vi "AddUser-Windows.vi"(7 "Login-UI.lvlib:PwdMgr.lvclass":refnum<class "PwdMgr.lvclass">, 8 "error in":errorcluster) -> (0 "error out":errorcluster)   [LabVIEW 2020, in "Login-UI.lvlib"]
uses:
  Login-UI.lvlib
  _Typedef/User-Role.ctl
  PwdMgr/PwdMgr.lvclass
  _Typedef/User-Info.ctl
panel:
  in  "Exit":bool
  in  "Save":bool
  in  "权  限":T1
  in  "密  码":string
  in  "用户名":string
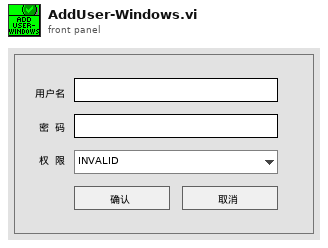
[diagram p1: front panel]
types:
  T1 = typedef "Login-UI.lvlib/User-Role.ctl" = enum16{"INVALID", "Operator", "Engineer", "Admin", "Anonymous"}
  T2 = enum32{"Invalid", "Standard", "Closed", "Hidden", "Minimized", "Maximized"}
  T3 = enum32{"invalid app kind", "Development System", "Run Time System", "Student Edition", "Embedded LabVIEW", "Evaluation", "Custom"}
  T4 = typedef "Login-UI.lvlib/User-Info.ctl" = cluster{"UserName":string, "Password":string, "Role":T1}
  T5 = cluster{"Core":cluster{"Current VI Reference":refnum<vi>, "Close Panel on Exit?":bool}, "Your Boolean data":bool, "Your string data":string, "Cluster":T4}
  T6 = typedef "eventvkey.ctl" = enum16{"ASCII", "Enter", "Return", "Shift", "Ctrl", "Alt", "Cmd", "Opt", "Caps", "NumLock", "Clear", "Break", "Up", "Down", "Left", "Right", "Insert", "Delete", "Home", "End", "PageUp", "PageDown", "Escape", "Help", "Pause", "ScrollLock", "F1", "F2", "F3", "F4", "F5", "F6", "F7", "F8", "F9", "F10", "F11", "F12", "F13", "F14", "F15", "F16", "F17", "F18", "F19", "F20", "F21", "F22", "F23", "F24", "Play", "VolumeUp", "VolumeDown", "Mute", "Two Byte Char"}
  T7 = cluster{"Current VI Reference":refnum<vi>, "Close Panel on Exit?":bool}
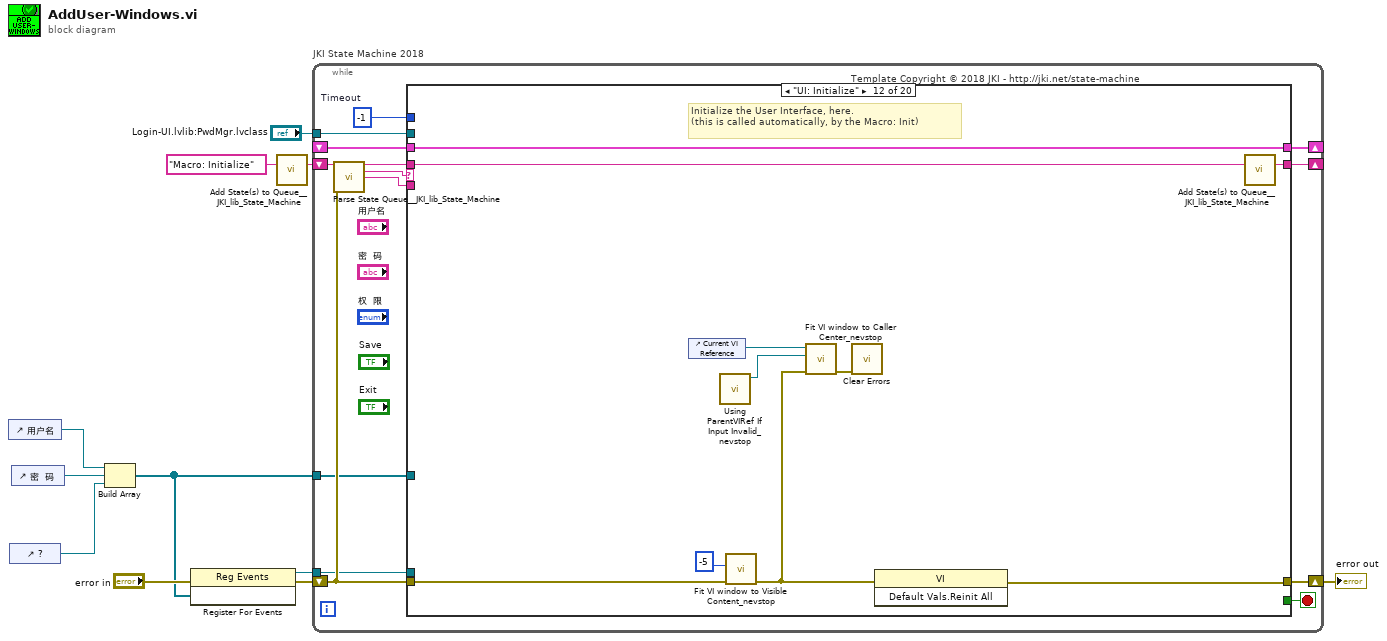
[diagram p0: block diagram]
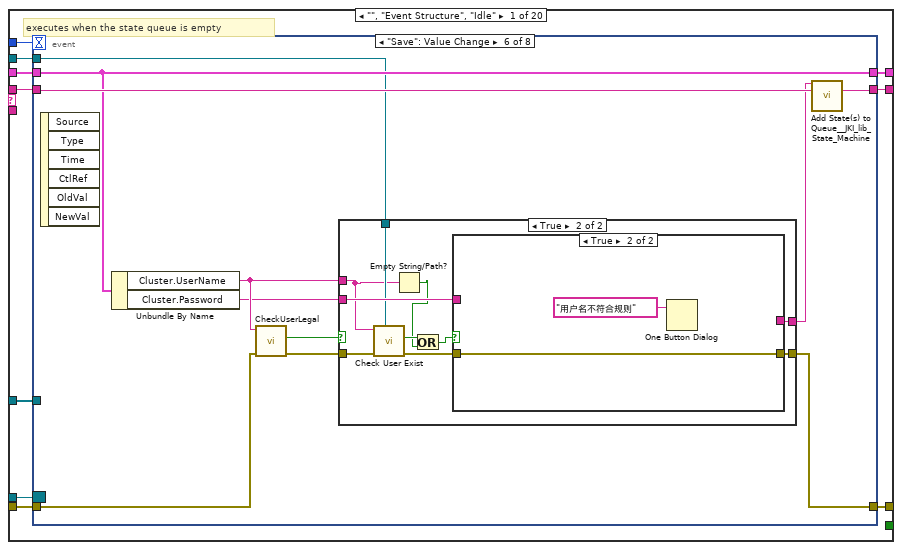
[diagram p2: hidden frame]
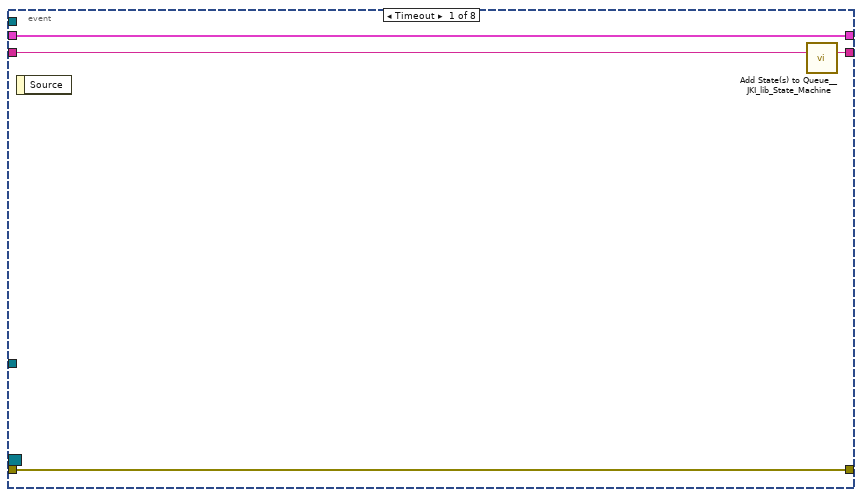
[diagram p3: hidden frame]
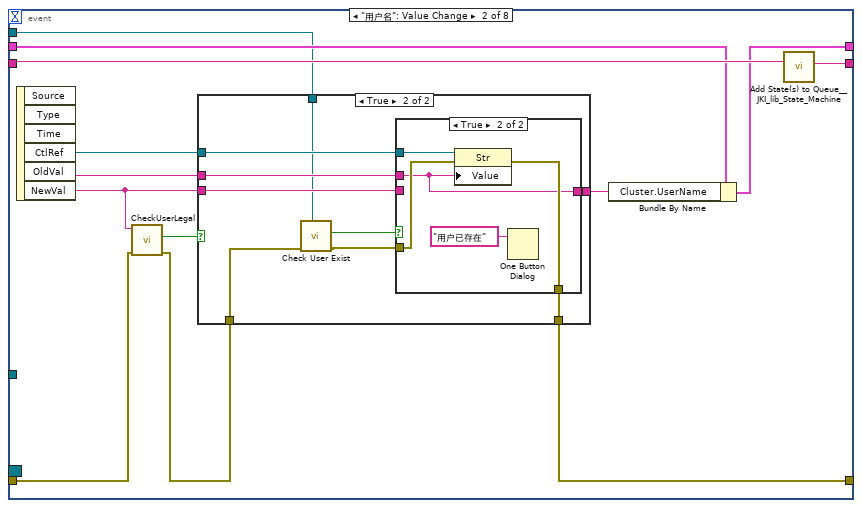
[diagram p4: hidden frame]
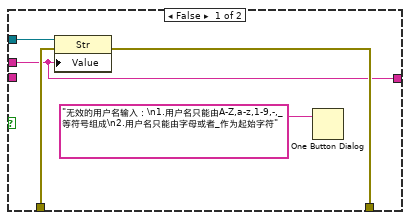
[diagram p5: hidden frame]
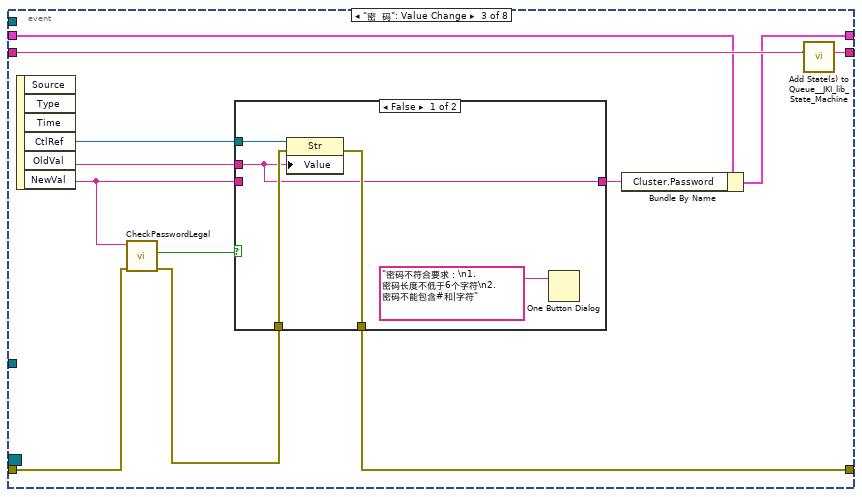
[diagram p7: hidden frame]
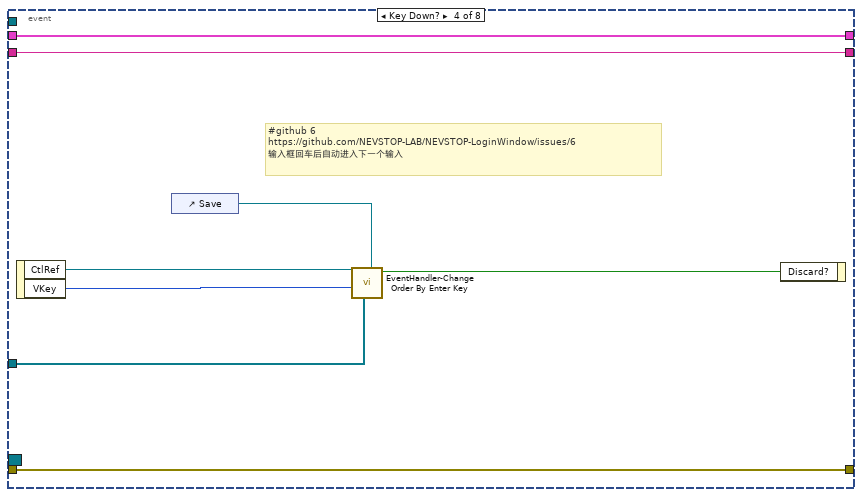
[diagram p9: hidden frame]
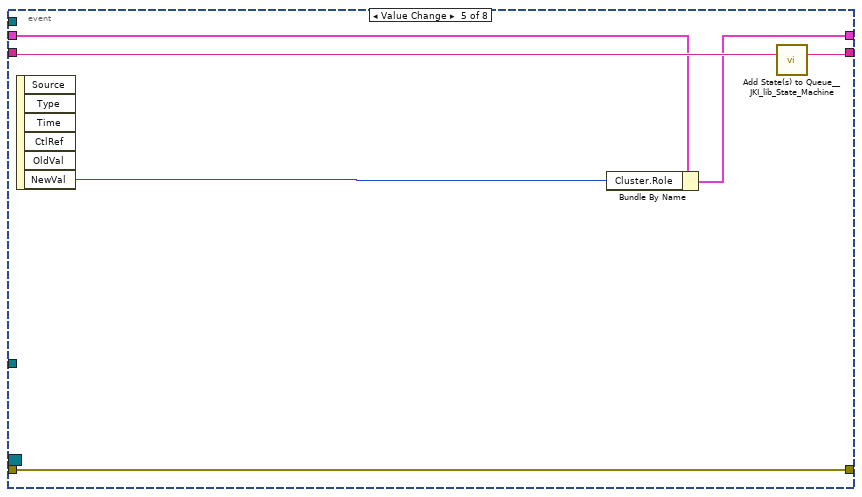
[diagram p10: hidden frame]
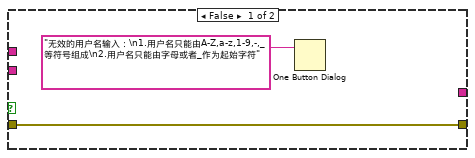
[diagram p11: hidden frame]
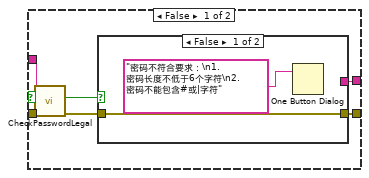
[diagram p12: hidden frame]
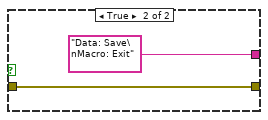
[diagram p13: hidden frame]
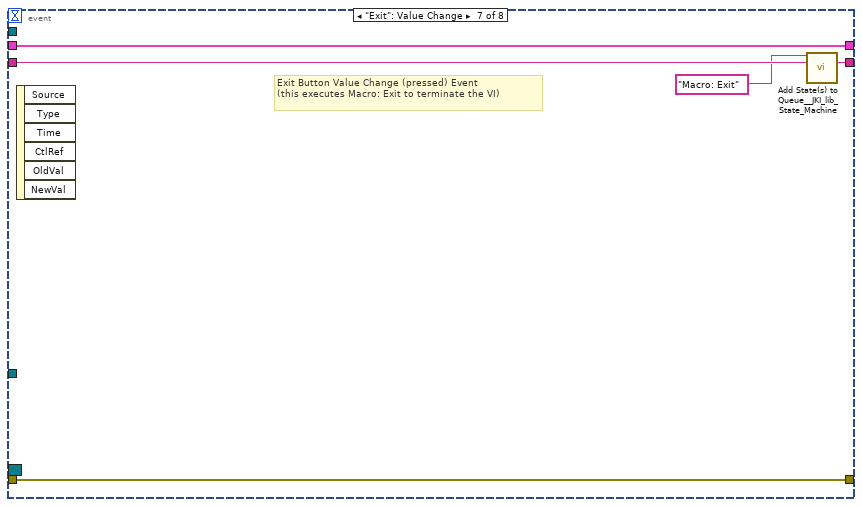
[diagram p14: hidden frame]
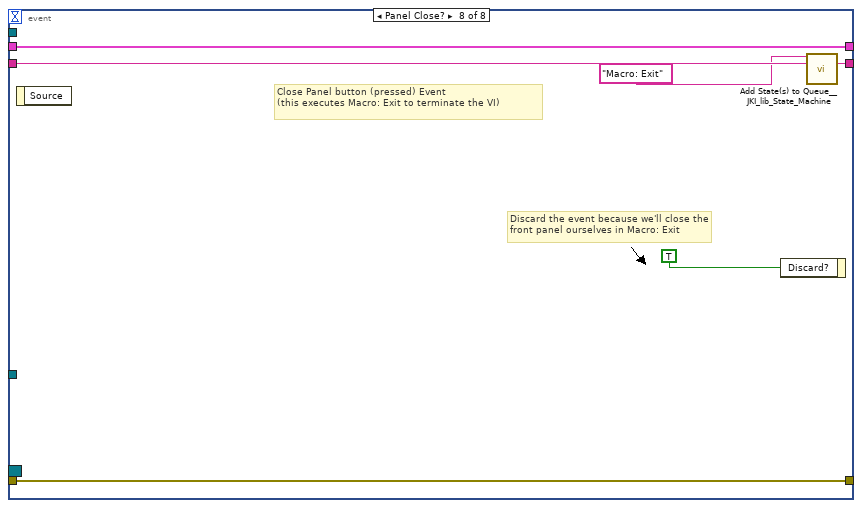
[diagram p15: hidden frame]
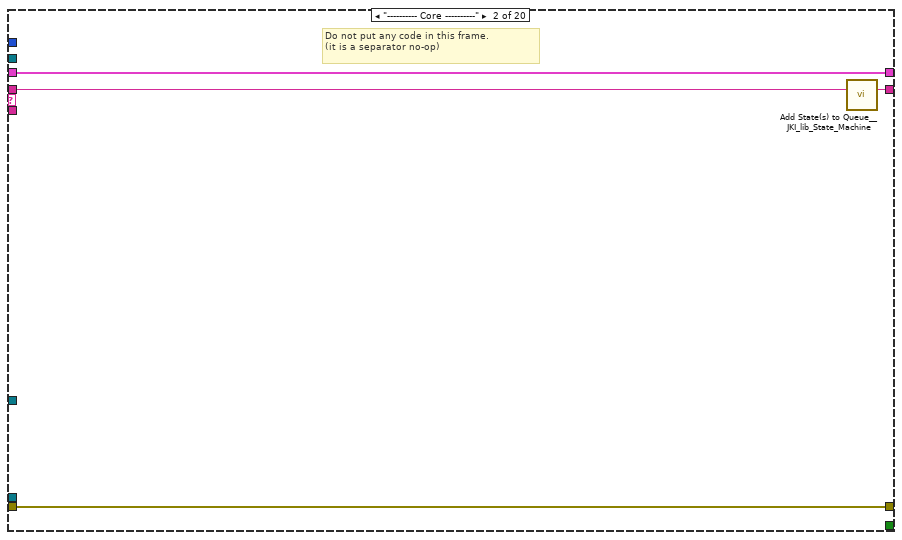
[diagram p16: hidden frame]
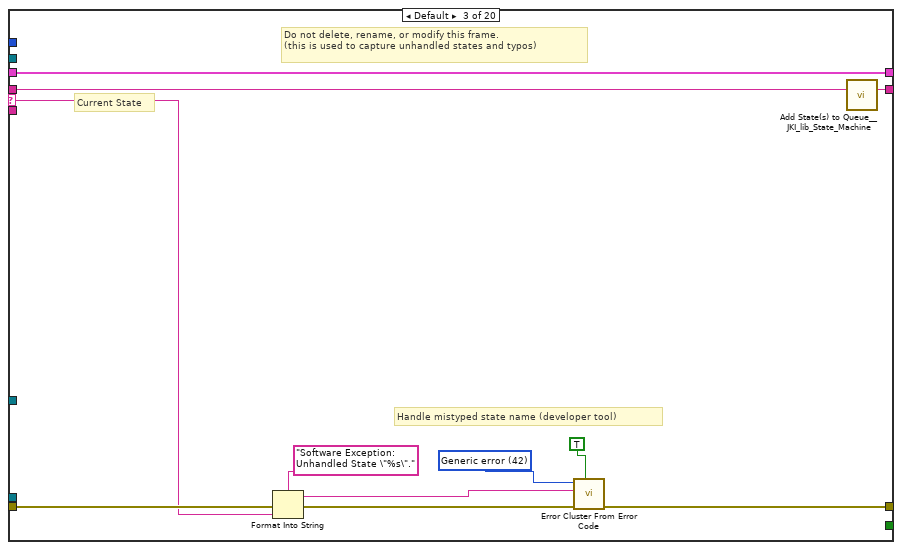
[diagram p17: hidden frame]
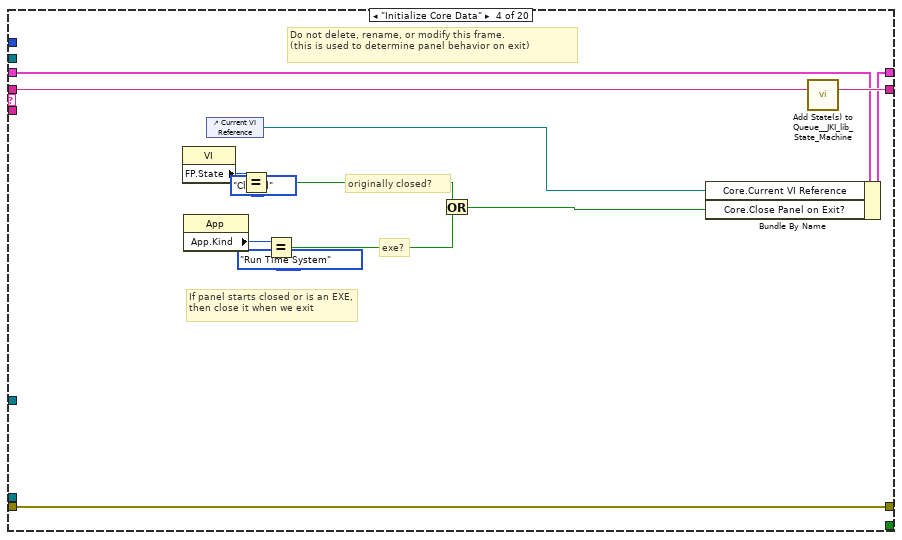
[diagram p18: hidden frame]
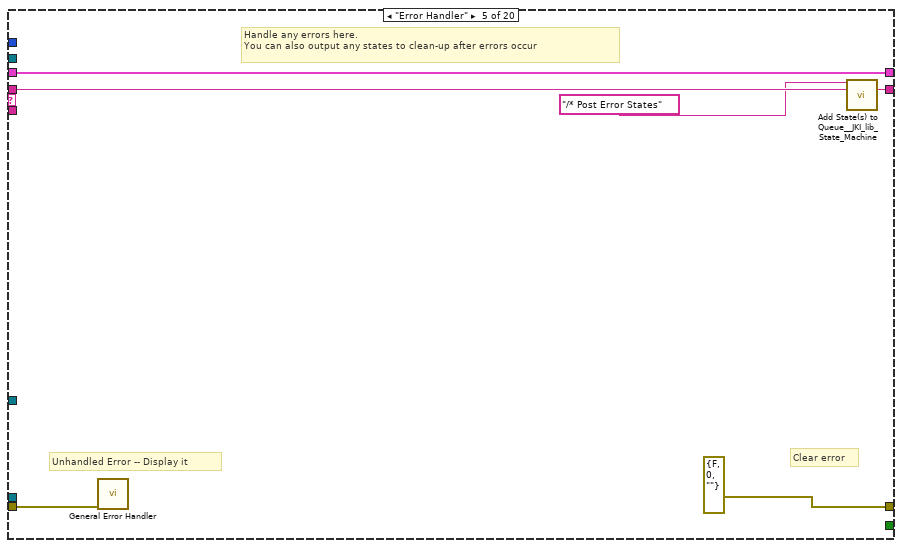
[diagram p19: hidden frame]
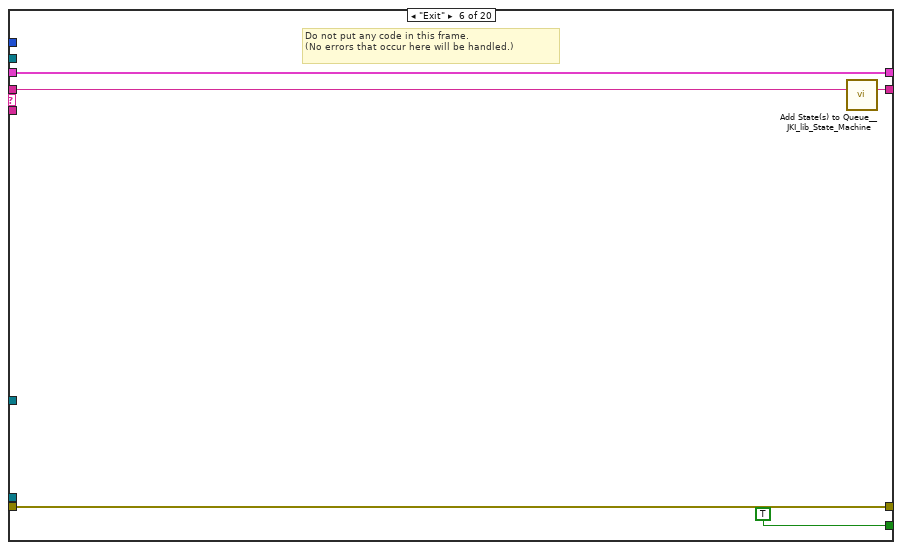
[diagram p20: hidden frame]
diagram:
  n1 = control-ref of="用户名"() -> (w2:refnum<vi>)
  n2 = control-ref of="?"() -> (w7:refnum<vi>)
  n3 = control-ref of="密  码"() -> (w3:refnum<vi>)
  n4 = Build Array(w2, w3, w7) -> (w4:refnum<vi>[])
  n5 = register-events(error in="error in", w4) -> (reference out=w5:refnum<event-registration>, error out=w6:errorcluster)  [unwired: 1 in]
  n6 = call <vilib>:"Add State(s) to Queue__JKI_lib_State_Machine.vi"("State(s) in (\"\")"="Macro: Initialize") -> ("States Out"=w11:string)  [unwired: 14 in]
  n7 = while "JKI State Machine 2018" {
    shift-right: [w18] -> _
    shift-left: _ -> [w17]
    shift-right: [w21] -> w8
    shift-left: w6 -> [w15]
    shift-right: [w20] -> _
    shift-left: w11 -> [w22]
    tunnel: w5 -> [w14]
    tunnel: w4 -> [w13]
    tunnel: "Login-UI.lvlib:PwdMgr.lvclass" -> [w12]
    stop <- w19 stop-if-true
    w16 = -1  # Timeout
    # "Template Copyright © 2018 JKI - http://jki.net/state-machine"
    n8 = call <vilib>:"Parse State Queue__JKI_lib_State_Machine.vi"("State Queue"=w22, "Error In (no error)"=w15) -> ("Remaining States"=w24:string, "Current State"=w25:string, "Arguments"=w23:string)  [unwired: 11 in]
    n9 = case shown="\"UI: Initialize\"" w25 {
      selector: w25 -> [_ _ w157 _ _ _ _ _ _ _ _ _ _ _ _ _ _ _ _ _]
      tunnel: w24 -> [w35 w156 w161 w180 w186 w191 w195 w203 w212 w219 w223 w233 w239 w250 w319 w324 w334 w338 w342 w346]
      tunnel: w23 -> [_ _ _ _ _ _ _ _ _ _ _ _ w234 w244 _ _ _ _ _ _]
      tunnel: w17 -> [w34 w153 w159 w173 w183 w189 w192 _ w210 w214 w220 w231 w237 w246 w316 w321 w331 w335 w339 w343]
      tunnel: [w33 w154 w163 w177 errorcluster {"status"=FALSE, "code"=0, "source"=""} ("error out") w188 w193 w200 w205 w215 w221 w228 w235 w247 w317 w322 w332 w336 w340 w344] -> w21
      tunnel: w15 -> [w32 w154 w162 w177 w182 w188 w193 w200 w207 w216 w221 w229 w236 w248 w317 w322 w332 w336 w340 w344]
      tunnel: [w29 w155 w160 w179 w185 w190 w194 w202 w213 w218 w222 w232 w238 w249 w318 w323 w333 w337 w341 w345] -> w20
      tunnel: [_ _ _ _ _ TRUE _ _ _ _ _ _ _ _ _ _ _ _ _ _] -> w19
      tunnel: [w31 w153 w159 w178 w183 w189 w192 w201 w210 w214 w220 w231 w237 w246 w316 w321 w331 w335 w339 w343] -> w18
      tunnel: w16 -> [w30 _ _ _ _ _ _ _ _ _ _ _ _ _ _ _ _ _ _ _]
      tunnel: w14 -> [w28 _ _ _ _ _ _ _ _ _ _ _ _ _ _ _ _ _ _ _]
      tunnel: w13 -> [w27 _ _ _ _ _ _ _ _ _ _ _ _ _ _ _ _ _ _ _]
      tunnel: w12 -> [w26 _ _ _ _ _ _ _ w204 _ _ _ _ _ _ _ _ _ _ _]
      frame "", "Event Structure", "Idle" {
        # "executes when the state queue is empty"
        n10 = event shown="[5] \"Save\": Value Change" {
          selector: w28 -> [_ _ _ _ _ _ _ _]
          dyn-events: _ -> [_ _ _ _ _ _ _ _]
          timeout: w30 -> [_ _ _ _ _ _ _ _]
          tunnel: w35 -> [w39 w48 w81 w94 w104 w116 w146 w152]
          tunnel: [w38 w49 w82 w94 w105 w117 w145 w151] -> w29
          tunnel: w34 -> [w36 w43 w76 w95 w102 w112 w143 w149]
          tunnel: [w37 w50 w83 w93 w106 w108 w144 w150] -> w33
          tunnel: w32 -> [w37 w45 w79 w93 w106 w109 w144 w150]
          tunnel: [w36 w41 w74 w95 w101 w112 w143 w149] -> w31
          tunnel: w27 -> [_ _ _ w97 _ _ _ _]
          tunnel: w26 -> [_ w40 _ _ _ w107 _ _]
          event Timeout {
            n11 = event-data() -> ()  [unwired: 1 in, 1 out]
            n12 = call <vilib>:"Add State(s) to Queue__JKI_lib_State_Machine.vi"("State(s) in (\"\")"=w39) -> ("States Out"=w38:string)  [unwired: 14 in]
          }
          event "用户名": Value Change {
            n13 = event-data() -> ("CtlRef"=w52:refnum<vi>, "OldVal"=w51:string, "NewVal"=w46:string)  [unwired: 1 in, 3 out]
            n14 = call "CheckUserLegal.vi"("error in (no error)"=w45, "Username"=w46) -> ("error out"=w44:errorcluster, "Legal?"=w47:bool)  [unwired: 8 in]
            n15 = case shown="True" w47 {
              tunnel: w52 -> [w56 w66]
              tunnel: w51 -> [w53 w65]
              tunnel: w46 -> [_ w60]
              tunnel: w44 -> [w55 w62]
              tunnel: [w54 w64] -> w50
              tunnel: [w53 w59] -> w42
              tunnel: w40 -> [_ w58]
              frame False {
                n16 = property class="Str"(reference=w56, error in=w55, "Value"=w53) -> (error out=w54:errorcluster)  [unwired: 1 out]
                n17 = One Button Dialog(message="无效的用户名输入：\n1.用户名只能由A-Z,a-z,1-9,-,_等符号组成\n2.用户名只能由字母或者_作为起始字符") -> ()  [unwired: 1 in, 1 out]
              }
              frame True {
                n18 = call-dynamic "Check User Exist.vi"("PwdMgr in"=w58, "Error in"=w62) -> ("Error out"=w61:errorcluster, "exist？"=w63:bool)  [unwired: 7 in, 1 out]
                n19 = case shown="True" w63 {
                  tunnel: w66 -> [_ w72]
                  tunnel: w65 -> [_ w69]
                  tunnel: w61 -> [w68 w71]
                  tunnel: [w68 w70] -> w64
                  tunnel: [w67 w69] -> w59
                  tunnel: w60 -> [w67 _]
                  frame False {
                  }
                  frame True {
                    n20 = property class="Str"(reference=w72, error in=w71, "Value"=w69) -> (error out=w70:errorcluster)  [unwired: 1 out]
                    n21 = One Button Dialog(message="用户已存在") -> ()  [unwired: 1 in, 1 out]
                  }
                }
              }
            }
            n22 = Bundle By Name(cluster=w43, "Cluster.UserName"=w42) -> (w41:T5)
            n23 = call <vilib>:"Add State(s) to Queue__JKI_lib_State_Machine.vi"("State(s) in (\"\")"=w48) -> ("States Out"=w49:string)  [unwired: 14 in]
          }
          event "密  码": Value Change {
            n24 = event-data() -> ("CtlRef"=w84:refnum<vi>, "OldVal"=w85:string, "NewVal"=w80:string)  [unwired: 1 in, 3 out]
            n25 = call "CheckPasswordLegal.vi"("error in (no error)"=w79, "Password"=w80) -> ("error out"=w78:errorcluster, "legal?"=w77:bool)  [unwired: 8 in]
            n26 = case shown="False" w77 {
              tunnel: w85 -> [w86 _]
              tunnel: w80 -> [_ w91]
              tunnel: [w89 w92] -> w83
              tunnel: w84 -> [w88 _]
              tunnel: w78 -> [w87 w92]
              tunnel: [w86 w91] -> w75
              frame False {
                n27 = property class="Str"(reference=w88, error in=w87, "Value"=w86) -> (error out=w89:errorcluster)  [unwired: 1 out]
                n28 = One Button Dialog(message="密码不符合要求：\n1.密码长度不低于6个字符\n2. 密码不能包含#和|字符") -> ()  [unwired: 1 in, 1 out]
              }
              frame True {
              }
            }
            n29 = Bundle By Name(cluster=w76, "Cluster.Password"=w75) -> (w74:T5)
            n30 = call <vilib>:"Add State(s) to Queue__JKI_lib_State_Machine.vi"("State(s) in (\"\")"=w81) -> ("States Out"=w82:string)  [unwired: 14 in]
          }
          event Key Down? {
            # "#github 6\nhttps://github.com/NEVSTOP-LAB/NEVSTOP-LoginWindow/issues/6\n输入框回车后自动进入下一个输入"
            n31 = event-data() -> ("CtlRef"=w100:refnum<vi>, "VKey"=w99:T6)  [unwired: 1 in]
            n32 = control-ref of="Save"() -> (w98:refnum<vi>)
            n33 = call "EventHandler-Change Order By Enter Key.vi"("Next Ctrl"=w98, "Controls for changing order"=w97, "VKey"=w99, "Event Control"=w100) -> ("Discard?"=w96:bool)  [unwired: 7 in]
            n34 = event-data("Discard?"=w96) -> ()  [unwired: 1 in, 1 out]
          }
          event Value Change {
            n35 = event-data() -> ("NewVal"=w103:T1)  [unwired: 1 in, 5 out]
            n36 = Bundle By Name(cluster=w102, "Cluster.Role"=w103) -> (w101:T5)
            n37 = call <vilib>:"Add State(s) to Queue__JKI_lib_State_Machine.vi"("State(s) in (\"\")"=w104) -> ("States Out"=w105:string)  [unwired: 14 in]
          }
          event "Save": Value Change {
            n38 = event-data() -> ()  [unwired: 1 in, 6 out]
            n39 = Unbundle By Name(w112) -> ("Cluster.UserName"=w114:string, "Cluster.Password"=w113:string)
            n40 = call "CheckUserLegal.vi"("error in (no error)"=w109, "Username"=w114) -> ("error out"=w110:errorcluster, "Legal?"=w115:bool)  [unwired: 8 in]
            n41 = case shown="True" w115 {
              tunnel: w114 -> [_ w122]
              tunnel: w113 -> [_ w128]
              tunnel: [_ w127] -> w111
              tunnel: w110 -> [w119 w126]
              tunnel: [w119 w124] -> w108
              tunnel: w107 -> [_ w123]
              frame False {
                n42 = One Button Dialog(message="无效的用户名输入：\n1.用户名只能由A-Z,a-z,1-9,-,_等符号组成\n2.用户名只能由字母或者_作为起始字符") -> ()  [unwired: 1 in, 1 out]
              }
              frame True {
                n43 = call-dynamic "Check User Exist.vi"("PwdMgr in"=w123, "Error in"=w126, "Username"=w122) -> ("Error out"=w125:errorcluster, "exist？"=w129:bool)  [unwired: 6 in, 1 out]
                n44 = Empty String/Path?(string/path=w122) -> (empty?=w120:bool)
                n45 = Or(x=w129, y=w120) -> (x .or. y?=w121:bool)
                n46 = case shown="True" w121 {
                  tunnel: w128 -> [w135 _]
                  tunnel: [w134 _] -> w127
                  tunnel: w125 -> [w133 w141]
                  tunnel: [w131 w141] -> w124
                  frame False {
                    n47 = call "CheckPasswordLegal.vi"("error in (no error)"=w133, "Password"=w135) -> ("error out"=w130:errorcluster, "legal?"=w132:bool)  [unwired: 8 in]
                    n48 = case shown="False" w132 {
                      tunnel: [_ "Data: Save\nMacro: Exit"] -> w134
                      tunnel: [w137 w138] -> w131
                      tunnel: w130 -> [w137 w138]
                      frame False {
                        n49 = One Button Dialog(message="密码不符合要求：\n1.密码长度不低于6个字符\n2. 密码不能包含#或|字符") -> ()  [unwired: 1 in, 1 out]
                      }
                      frame True {
                      }
                    }
                  }
                  frame True {
                    n50 = One Button Dialog(message="用户名不符合规则") -> ()  [unwired: 1 in, 1 out]
                  }
                }
              }
            }
            n51 = call <vilib>:"Add State(s) to Queue__JKI_lib_State_Machine.vi"("State(s) in Front (\"\")"=w111, "State(s) in (\"\")"=w116) -> ("States Out"=w117:string)  [unwired: 13 in]
          }
          event "Exit": Value Change {
            # "Exit Button Value Change (pressed) Event\n(this executes Macro: Exit to terminate the VI)"
            n52 = event-data() -> ()  [unwired: 1 in, 6 out]
            n53 = call <vilib>:"Add State(s) to Queue__JKI_lib_State_Machine.vi"("State(s) in Front (\"\")"="Macro: Exit", "State(s) in (\"\")"=w146) -> ("States Out"=w145:string)  [unwired: 13 in]
          }
          event Panel Close? {
            # "Discard the event because we'll close the front panel ourselves in Macro: Exit"
            # "Close Panel button (pressed) Event\n(this executes Macro: Exit to terminate the VI)"
            n54 = event-data() -> ()  [unwired: 1 in, 1 out]
            n55 = event-data("Discard?"=TRUE) -> ()  [unwired: 1 in, 1 out]
            n56 = call <vilib>:"Add State(s) to Queue__JKI_lib_State_Machine.vi"("State(s) in Front (\"\")"="Macro: Exit", "State(s) in (\"\")"=w152) -> ("States Out"=w151:string)  [unwired: 13 in]
          }
        }
      }
      frame "---------- Core ----------" {
        # "Do not put any code in this frame.\n(it is a separator no-op)"
        n57 = call <vilib>:"Add State(s) to Queue__JKI_lib_State_Machine.vi"("State(s) in (\"\")"=w156) -> ("States Out"=w155:string)  [unwired: 14 in]
      }
      frame Default {
        w166 = 42 items=["No error", "Argument error", "Memory is full", "Out of zone", "End of file", "File already open", "Generic file I/O error", "File not found", "File permission error", "Disk is full", "Duplicate path", "Too many files open", "System feature not enabled", "Resource file not found", "Cannot add resource", "Resource not found", "Image not found", "Image memory error", "Pen does not exist", "Config type invalid", "Config token not found", "Config parse error", "Config memory error", "Bad external code format", "Bad external code offset", "External code not present", "Null window", "Destroy window error", "Null menu", "Print aborted", "Bad print record", "Print driver error", "Windows error during printing", "Memory error during printing", "Print dialog error", "Generic print error", "Invalid device refnum", "Device not found", "Device parameter error", "Device unit error", "Cannot open device", "Device call aborted", "Generic error", "Cancelled by user", "Object ID too low", "Object ID too high", "Object not in heap", "Unknown heap", "Unknown object (invalid DefProc)", "Unknown object (DefProc not in table)", "Message out of range", "Invalid (null) method", "Unknown message", "Manager call not supported", "Bad address", "Network operation in progress", "Network operation timed out", "Connection is busy", "Network attribute not supported", "Network error", "Address in use", "System out of memory", "Connection aborted", "Connection refused", "Not connected", "Already connected", "Connection closed", "Initialization error (interapplication manager)", "Bad occurrence", "Wait on unbound occurrence handler", "Occurrence queue overflow", "Datalog type conflict", "Unused", "Unrecognized type (interapplication manager)", "Memory corrupt", "Failed to make temporary DLL", "Old CIN version", "Drag socket not found", "Failed to load drop-object", "Failed to register OLE object", "Failed to release OLE object", "Format specifier type mismatch", "Unknown format specifier", "Too few format specifiers", "Too many format specifiers", "Scan failed", "Newer CIN version", "Error converting to variant", "Runtime menu error", "Password tampered", "Variant attribute not found", "Incompatible variant data type", "Event data is not available", "Event Store is not present", "Occurrence is not found", "Event Queue is not created", "Event info is not available", "Refnum passed is NULL", "Error retrieving Class GUID", "Error retrieving CoClass GUID", "Error retrieving TypeLib GUID.", "Bad built application magic bytes.", "Specific driver is different from the specific driver associated with the Logical Name.", "There is no session opened to the class driver.", "Max Error", "MAX - Error with config objects", "MAX - Error loading configuration", "MAX - Group not supported"]
        # "Current State"
        # "Do not delete, rename, or modify this frame.\n(this is used to capture unhandled states and typos)"
        # "Handle mistyped state name (developer tool)"
        n58 = Format Into String(format string="Software Exception: Unhandled State \"%s\"." ("message"), error in=w162, w157) -> (resulting string=w165:string, error out=w164:errorcluster)  [unwired: 1 in]
        n59 = call <vilib>:"Error Cluster From Error Code.vi"("show call chain? (False)"=TRUE, "error in (no error)"=w164, "error message (\"\")"=w165, "error code (0)"=w166) -> ("error out"=w163:errorcluster)  [unwired: 5 in]
        n60 = call <vilib>:"Add State(s) to Queue__JKI_lib_State_Machine.vi"("State(s) in (\"\")"=w161) -> ("States Out"=w160:string)  [unwired: 14 in]
      }
      frame "Initialize Core Data" {
        # "Do not delete, rename, or modify this frame.\n(this is used to determine panel behavior on exit)"
        # "originally closed?"
        # "exe?"
        # "If panel starts closed or is an EXE, then close it when we exit"
        n61 = property class="VI"() -> ("FP.State"=w170:T2)  [unwired: 2 in, 2 out]
        n62 = property class="App"() -> ("App.Kind"=w176:T3)  [unwired: 2 in, 2 out]
        n63 = control-ref of="Current VI Reference"() -> (w171:refnum<vi>)
        n64 = Equal?(x=w170, y=T2."Closed" ("Front Panel Window:State")) -> (x = y?=w168:bool)
        n65 = Equal?(x=w176, y=T3."Run Time System" ("Application:Kind")) -> (x = y?=w174:bool)
        n66 = Or(x=w168, y=w174) -> (x .or. y?=w172:bool)
        n67 = Bundle By Name(cluster=w173, "Core.Current VI Reference"=w171, "Core.Close Panel on Exit?"=w172) -> (w178:T5)
        n68 = call <vilib>:"Add State(s) to Queue__JKI_lib_State_Machine.vi"("State(s) in (\"\")"=w180) -> ("States Out"=w179:string)  [unwired: 14 in]
      }
      frame "Error Handler" {
        # "Unhandled Error -- Display it"
        # "Handle any errors here.\nYou can also output any states to clean-up after errors occur"
        # "Clear error"
        n69 = call <vilib>:"General Error Handler.vi"("error in (no error)"=w182) -> ()  [unwired: 10 in, 5 out]
        n70 = call <vilib>:"Add State(s) to Queue__JKI_lib_State_Machine.vi"("State(s) in Front (\"\")"="/* Post Error States", "State(s) in (\"\")"=w186) -> ("States Out"=w185:string)  [unwired: 13 in]
      }
      frame "Exit" {
        # "Do not put any code in this frame.\n(No errors that occur here will be handled.)"
        n71 = call <vilib>:"Add State(s) to Queue__JKI_lib_State_Machine.vi"("State(s) in (\"\")"=w191) -> ("States Out"=w190:string)  [unwired: 14 in]
      }
      frame "---------- Data ----------" {
        # "Do not put any code in this frame.\n(It is a separator no-op. You can make a copy of this frame to create a new Data frame)"
        n72 = call <vilib>:"Add State(s) to Queue__JKI_lib_State_Machine.vi"("State(s) in (\"\")"=w195) -> ("States Out"=w194:string)  [unwired: 14 in]
      }
      frame "Data: Initialize" {
        w197 = T7 {"Current VI Reference"=refnum, "Close Panel on Exit?"=FALSE}  # Core
        w199 = TRUE  # Your Boolean data
        w198 = ""  # Your string data
        # "do not delete - used by framework"
        # "Add new data here."
        # "Data names and types of shift register data are defined by this bundle."
        # "Initialize the shift-register data, here.\n(data names are defined by what you wire into the bundle function)"
        n73 = Bundle("Core"=w197, "Your Boolean data"=w199, "Your string data"=w198, "Cluster"=T4 {"UserName"="", "Password"="", "Role"=enum."INVALID"}) -> (w201:T5)  [unwired: 1 in]
        n74 = call <vilib>:"Add State(s) to Queue__JKI_lib_State_Machine.vi"("State(s) in (\"\")"=w203) -> ("States Out"=w202:string)  [unwired: 14 in]
      }
      frame "Data: Save" {
        n75 = Unbundle By Name(w210) -> ("Cluster"=w209:T4)
        n76 = call-dynamic "List Users.vi"("PwdMgr in"=w204, "error in (no error)"=w207) -> ("error out"=w206:errorcluster, "Array"=w211:T4[])  [unwired: 8 in]
        n77 = Build Array (concatenate)(w211, w209) -> (w208:T4[])
        n78 = call-dynamic "Save Users.vi"("PwdMgr in"=w204, "error in (no error)"=w206, "Array"=w208) -> ("error out"=w205:errorcluster)  [unwired: 8 in]
        n79 = call <vilib>:"Add State(s) to Queue__JKI_lib_State_Machine.vi"("State(s) in (\"\")"=w212) -> ("States Out"=w213:string)  [unwired: 14 in]
      }
      frame "Data: Cleanup" {
        # "Cleanup any data and references, here.\n(this is called automatically, by the Macro: Exit)"
        n80 = Unbundle By Name(w214) -> ("Core.Current VI Reference"=w217:refnum<vi>)
        n81 = Close Reference(reference=w217, error in (no error)=w216) -> (error out=w215:errorcluster)
        n82 = call <vilib>:"Add State(s) to Queue__JKI_lib_State_Machine.vi"("State(s) in (\"\")"=w219) -> ("States Out"=w218:string)  [unwired: 14 in]
      }
      frame "---------- UI ----------" {
        # "Do not put any code in this frame.\n(It is a separator no-op. You can make a copy of this frame to create a new UI frame)"
        n83 = call <vilib>:"Add State(s) to Queue__JKI_lib_State_Machine.vi"("State(s) in (\"\")"=w223) -> ("States Out"=w222:string)  [unwired: 14 in]
      }
      frame "UI: Initialize" {
        # "Initialize the User Interface, here.\n(this is called automatically, by the Macro: Init)"
        n84 = control-ref of="Current VI Reference"() -> (w226:refnum<vi>)
        n85 = call <userlib>:"Using ParentVIRef If Input Invalid_nevstop.vi"() -> ("VI Ref"=w225:refnum<vi>)  [unwired: 6 in, 1 out]
        n86 = call <userlib>:"Fit VI window to Visible Content_nevstop.vi"("error in (no error)"=w229, "border spacing (2 px)"=-5) -> ("error out"=w224:errorcluster)  [unwired: 4 in, 1 out]
        n87 = call <userlib>:"Fit VI window to Caller Center_nevstop.vi"("Error In"=w224, "Background VI Ref (Callee's Caller)"=w225, "VI Ref (calling VI)"=w226) -> ("Error Out"=w227:errorcluster)  [unwired: 3 in, 1 out]
        n88 = call <vilib>:"Clear Errors.vi"("error in (no error)"=w227) -> ()  [unwired: 5 in, 2 out]
        n89 = invoke class="VI" method="Default Vals.Reinit All"(error in=w224) -> (error out=w228:errorcluster)  [unwired: 2 in, 2 out]
        n90 = call <vilib>:"Add State(s) to Queue__JKI_lib_State_Machine.vi"("State(s) in (\"\")"=w233) -> ("States Out"=w232:string)  [unwired: 14 in]
      }
      frame "UI: Cursor Set" {
        # "Argument"
        # "Set and Unset Cursor Busy.\n(Usage: \"UI: Cursor Set >> Busy|Idle\")"
        n91 = case shown="\"Idle\", Default" w234 {
          tunnel: w236 -> [w241 w243]
          tunnel: [w240 w242] -> w235
          frame "Idle", Default {
            n92 = call <vilib>:"Unset Busy.vi"("error in (no error)"=w241) -> ("error out"=w240:errorcluster)  [unwired: 10 in]
          }
          frame "Busy" {
            n93 = call <vilib>:"Set Busy.vi"("error in (no error)"=w243) -> ("error out"=w242:errorcluster)  [unwired: 9 in, 1 out]
          }
        }
        n94 = call <vilib>:"Add State(s) to Queue__JKI_lib_State_Machine.vi"("State(s) in (\"\")"=w239) -> ("States Out"=w238:string)  [unwired: 14 in]
      }
      frame "UI: Front Panel State" {
        # "Argument"
        # "Set Front Panel Open or Closed\n(Usage: \"UI: Front Panel State >> Open|Close\")"
        n95 = Unbundle By Name(w246) -> ("Core.Current VI Reference"=w245:refnum<vi>)
        n96 = case shown="\"Minimize\", \"Minimized\"" w244 {
          tunnel: w248 -> [w256 w271 w282 w295 w308]
          tunnel: [w258 w272 w284 w297 w310] -> w247
          tunnel: w245 -> [w257 w269 w283 w296 w309]
          frame "Open", "Standard", Default {
            w251 = T2."Standard" ("State")
            n97 = property class="VI"(reference=w257, error in=w256) -> (reference out=w254:refnum<vi>, error out=w255:errorcluster, "FP.State"=w253:T2)
            n98 = Not Equal?(x=w253, y=w251) -> (x != y?=w252:bool)
            n99 = case shown="True" w252 {
              tunnel: [w262 w264] -> w258
              tunnel: w255 -> [w261 w264]
              tunnel: w254 -> [w260 _]
              tunnel: w251 -> [w259 _]
              frame True {
                n100 = invoke class="VI" method="FP.Open"(reference=w260, error in=w261, "Activate"=TRUE, "State"=w259) -> (error out=w262:errorcluster)  [unwired: 1 in, 4 out]
              }
              frame False {
              }
            }
          }
          frame "Close", "Closed" {
            n101 = property class="VI"(reference=w269, error in=w271) -> (reference out=w268:refnum<vi>, error out=w270:errorcluster, "FP.State"=w266:T2)
            n102 = Not Equal?(x=w266, y=T2."Closed" ("Front Panel Window:State")) -> (x != y?=w265:bool)
            n103 = case shown="True" w265 {
              tunnel: [w273 w276] -> w272
              tunnel: w270 -> [w273 w275]
              tunnel: w268 -> [_ w274]
              frame False {
              }
              frame True {
                n104 = invoke class="VI" method="FP.Close"(reference=w274, error in=w275) -> (error out=w276:errorcluster)  [unwired: 1 in, 2 out]
              }
            }
          }
          frame "Hidden", "Hide" {
            w277 = T2."Hidden" ("State")
            n105 = property class="VI"(reference=w283, error in=w282) -> (reference out=w280:refnum<vi>, error out=w281:errorcluster, "FP.State"=w279:T2)
            n106 = Not Equal?(x=w279, y=w277) -> (x != y?=w278:bool)
            n107 = case shown="True" w278 {
              tunnel: [w288 w289] -> w284
              tunnel: w281 -> [w287 w289]
              tunnel: w280 -> [w286 _]
              tunnel: w277 -> [w285 _]
              frame True {
                n108 = invoke class="VI" method="FP.Open"(reference=w286, error in=w287, "State"=w285) -> (error out=w288:errorcluster)  [unwired: 2 in, 4 out]
              }
              frame False {
              }
            }
          }
          frame "Minimize", "Minimized" {
            w290 = T2."Minimized" ("State")
            n109 = property class="VI"(reference=w296, error in=w295) -> (reference out=w293:refnum<vi>, error out=w294:errorcluster, "FP.State"=w292:T2)
            n110 = Not Equal?(x=w292, y=w290) -> (x != y?=w291:bool)
            n111 = case shown="True" w291 {
              tunnel: [w301 w302] -> w297
              tunnel: w294 -> [w300 w302]
              tunnel: w293 -> [w299 _]
              tunnel: w290 -> [w298 _]
              frame True {
                n112 = invoke class="VI" method="FP.Open"(reference=w299, error in=w300, "State"=w298) -> (error out=w301:errorcluster)  [unwired: 2 in, 4 out]
              }
              frame False {
              }
            }
          }
          frame "Maximize", "Maximized" {
            w303 = T2."Maximized" ("State")
            n113 = property class="VI"(reference=w309, error in=w308) -> (reference out=w306:refnum<vi>, error out=w307:errorcluster, "FP.State"=w305:T2)
            n114 = Not Equal?(x=w305, y=w303) -> (x != y?=w304:bool)
            n115 = case shown="True" w304 {
              tunnel: [w314 w315] -> w310
              tunnel: w307 -> [w313 w315]
              tunnel: w306 -> [w312 _]
              tunnel: w303 -> [w311 _]
              frame True {
                n116 = invoke class="VI" method="FP.Open"(reference=w312, error in=w313, "State"=w311) -> (error out=w314:errorcluster)  [unwired: 2 in, 4 out]
              }
              frame False {
              }
            }
          }
        }
        n117 = call <vilib>:"Add State(s) to Queue__JKI_lib_State_Machine.vi"("State(s) in (\"\")"=w250) -> ("States Out"=w249:string)  [unwired: 14 in]
      }
      frame "---------- Macro ----------" {
        # "Do not put any code in this frame.\n(It is a separator no-op. You can make a copy of this frame to create a new Macro frame)"
        n118 = call <vilib>:"Add State(s) to Queue__JKI_lib_State_Machine.vi"("State(s) in (\"\")"=w319) -> ("States Out"=w318:string)  [unwired: 14 in]
      }
      frame "Macro: Initialize" {
        w320 = "Data: Initialize\nInitialize Core Data\nUI: Initialize\nUI: Front Panel State >> Open"  # Data: Initialize Initialize Core Data UI: Initialize UI: Front Panel State >> Open
        # "Initialization Macro\n(This is called once, when the VI starts)"
        n119 = call <vilib>:"Add State(s) to Queue__JKI_lib_State_Machine.vi"("State(s) in Front (\"\")"=w320, "State(s) in (\"\")"=w324) -> ("States Out"=w323:string)  [unwired: 13 in]
      }
      frame "Macro: Exit" {
        # "Exit Macro\n(This is called once, when the VI exits)"
        n120 = Unbundle By Name(w331) -> ("Core.Close Panel on Exit?"=w330:bool)
        n121 = Select(t="UI: Front Panel State >> Close", s=w330, f="") -> (s? t:f=w327:string)
        n122 = call <vilib>:"Add State(s) to Queue__JKI_lib_State_Machine.vi"("State(s) in (\"\")"=w327, "State(s) at Back (\"\")"="Data: Cleanup\nExit") -> ("States Out"=w325:string)  [unwired: 13 in]
        n123 = call <vilib>:"Add State(s) to Queue__JKI_lib_State_Machine.vi"("State(s) in Front (\"\")"=w325, "State(s) in (\"\")"=w334) -> ("States Out"=w333:string)  [unwired: 13 in]
      }
      frame "---------- New Category ----------" {
        # "Template Separator\n(You can make a copy of, or modify, this frame)"
        n124 = call <vilib>:"Add State(s) to Queue__JKI_lib_State_Machine.vi"("State(s) in (\"\")"=w338) -> ("States Out"=w337:string)  [unwired: 14 in]
      }
      frame "New Category: 1" {
        # "Your code here.\n(You can make a copy of, or modify, this frame)"
        n125 = call <vilib>:"Add State(s) to Queue__JKI_lib_State_Machine.vi"("State(s) in (\"\")"=w342) -> ("States Out"=w341:string)  [unwired: 14 in]
      }
      frame "New Category: 2" {
        # "Your code here.\n(You can make a copy of, or modify, this frame)"
        n126 = call <vilib>:"Add State(s) to Queue__JKI_lib_State_Machine.vi"("State(s) in (\"\")"=w346) -> ("States Out"=w345:string)  [unwired: 14 in]
      }
    }
  }
  "error out" <- w8
